vi "FlipRect.vi"(8 "错误输入":errorcluster, 9 "模式":enum16{"水平", "垂直"}(ring), 11 "rect":T1 caption="矩形") -> (0 "错误输出":errorcluster, 3 "flipped rect":T1 caption="翻转矩形")   [LabVIEW 2011, in "Rect Tools.lvlib"]
uses:
  Rect Tools.lvlib
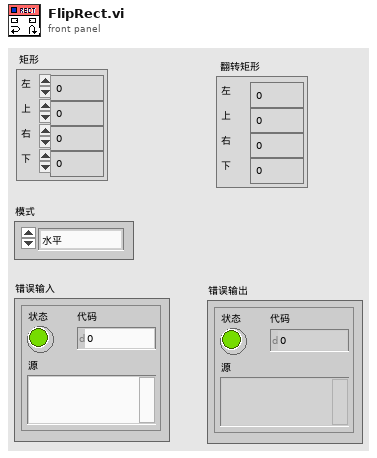
[diagram p1: front panel]
types:
  T1 = cluster{"left":i16, "top":i16, "right":i16, "bottom":i16}
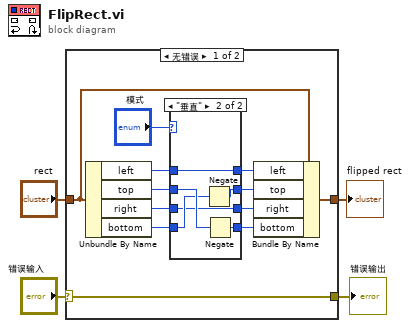
[diagram p0: block diagram]
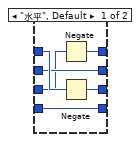
[diagram p2: hidden frame]
diagram:
  n1 = case shown="无错误" "错误输入" {
    selector: "错误输入" -> [w7 w30]
    tunnel: [w7 w30] -> w3
    tunnel: "rect" -> [w6 w29]
    tunnel: [w5 w29] -> w1
    frame No Error {
      n2 = Unbundle By Name(w6) -> ("left"=w11:i16, "top"=w14:i16, "right"=w9:i16, "bottom"=w13:i16)
      n3 = case shown="\"垂直\"" "模式" {
        tunnel: [w21 w23] -> w16
        tunnel: [w19 w24] -> w15
        tunnel: w14 -> [w21 w28]
        tunnel: w13 -> [w19 w27]
        tunnel: [w17 w26] -> w12
        tunnel: w11 -> [w22 w26]
        tunnel: [w18 w25] -> w10
        tunnel: w9 -> [w20 w25]
        frame "水平", Default {
          n4 = Negate(x=w20) -> (-x=w17:i16)
          n5 = Negate(x=w22) -> (-x=w18:i16)
        }
        frame "垂直" {
          n6 = Negate(x=w27) -> (-x=w23:i16)
          n7 = Negate(x=w28) -> (-x=w24:i16)
        }
      }
      n8 = Bundle By Name(cluster=w6, "left"=w12, "top"=w16, "right"=w10, "bottom"=w15) -> (w5:T1)
    }
    frame Error {
    }
  }
  "错误输出" <- w3
  "flipped rect" <- w1
